vi "Read Single Point.vi"(0 "VISA resource name":refnum<visa-resource-name>, 11 "error in (no error)":errorcluster) -> (4 "VISA resource name out":refnum<visa-resource-name>, 6 "Measurement Data":dbl, 15 "error out":errorcluster)   [LabVIEW 2015, in "Keithley 27XX.lvlib"]
doc: "This VI is used to initiate a single reading and transfer that reading over the bus.\n\nThis VI will only return the first value read.\n\nNote:\nTo read multiple data elements, use one of the read multiple instances of this VI."
uses:
  Keithley 27XX.lvlib
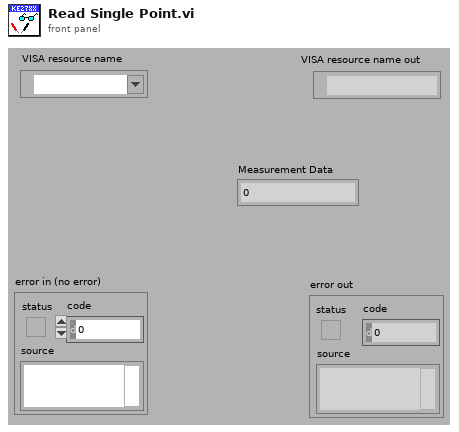
[diagram p1: front panel]
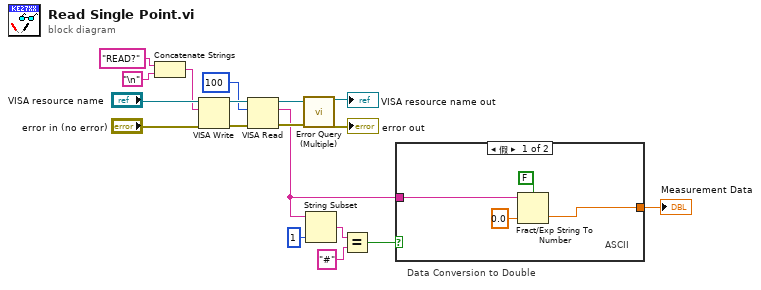
[diagram p0: block diagram]
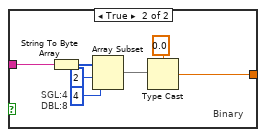
[diagram p2: hidden frame]
diagram:
  # "Data Conversion to Double"
  n1 = Concatenate Strings("READ?" ("write buffer"), "\n") -> (w3:string)
  n2 = VISA Write(VISA resource name="VISA resource name", write buffer=w3, error in (no error)="error in (no error)") -> (VISA resource name out=w18:refnum<visa-resource-name>, error out=w17:errorcluster)  [unwired: 1 out]
  n3 = VISA Read(VISA resource name=w18, byte count=u32 100, error in (no error)=w17) -> (VISA resource name out=w15:refnum<visa-resource-name>, read buffer=w9:string, error out=w14:errorcluster)  [unwired: 1 out]
  n4 = call "Error Query (Multiple).vi"("VISA resource name"=w15, "error in (no error)"=w14) -> ("VISA resource name out"=→"VISA resource name out":refnum<visa-resource-name>, "error out"=→"error out":errorcluster)  [unwired: 10 in, 2 out]
  n5 = String Subset(string=w9, length (rest)=1 ("length (rest)")) -> (substring=w11:string)  [unwired: 1 in]
  n6 = Equal?(x=w11, y="#") -> (x = y?=w8:bool)
  n7 = case shown="假" w8 {
    tunnel: w9 -> [w22 w24]
    tunnel: [w21 w23] -> w1
    frame False {
      # "ASCII"
      n8 = Fract/Exp String To Number(use system decimal point (T)=FALSE, string=w22, default (0 dbl)=sgl 0.0 ("default (0 DBL)")) -> (number=w21:sgl)  [unwired: 1 in, 1 out]
    }
    frame True {
      # "SGL:4\nDBL:8"
      # "Binary"
      n9 = String To Byte Array(string=w24) -> (unsigned byte array=w29:u8[])
      n10 = Array Subset(array=w29, index=2, length=4) -> (w26:u8[])
      n11 = Type Cast(type=sgl 0.0, x=w26) -> (*(type *) &x=w23:sgl)
    }
  }
  "Measurement Data" <- w1
